vi "Configure Multi Eval Meas List Segment Bandwidth Part.vi"(0 "VISA resource name":refnum<visa-resource-name>, 1 "BWP (0)":i32, 2 "Cyclic Prefix (Normal)":i32(ring) items=["Normal", "Extended"], 3 "Start RB (0)":i32, 5 "Instance (1)":T2=1, 7 "Segment (1)":i32=1, 9 "CC (1)":T1=1, 11 "error in (no error)":errorcluster, 12 "Subcarrier Spacing (30 kHz)":i32(ring)=1 items=["15 kHz", "30 kHz", "60 kHz"], 13 "Number RB (66)":i32=66) -> (4 "VISA resource name out":refnum<visa-resource-name>, 15 "error out":errorcluster)   [LabVIEW 2020, in "Rohde&Schwarz CMWXP NR FR1 Measurement.lvlib"]
doc: "Configures basic properties of the <BWP> on carrier <cc> in segment <no>.\n\nAttribute:\nRSCMWXPNRFR1M_ATTR_MULTI_EVAL_MEAS_LIST_SEGMENT_BANDWIDTH_PART\n\nRemote-control command:\nCONFigure:NRSub:MEAS<i>:LIST:SEGMent<no>[:CC<cc>]:BWPart"
uses:
  <instrlib>/Rohde&Schwarz CMWXP NR FR1 Measurement/Rohde&Schwarz CMWXP NR FR1 Measurement.lvlib
  <instrlib>/Rohde&Schwarz CMWXP NR FR1 Measurement/Private/_Instance.ctl
  <instrlib>/Rohde&Schwarz CMWXP NR FR1 Measurement/Private/_Carrier Component.ctl
  <instrlib>/Rohde&Schwarz CMWXP NR FR1 Measurement/Private/rsidr_core.llb/rsidr_core.lvlib
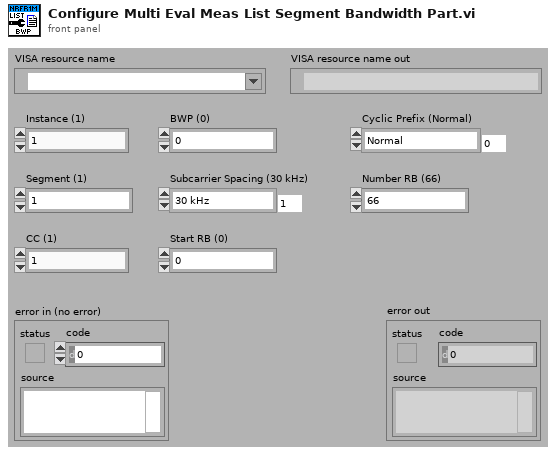
[diagram p1: front panel]
types:
  T1 = typedef "Rohde&Schwarz CMWXP NR FR1 Measurement.lvlib/_Carrier Component.ctl" = i32
  T2 = typedef "Rohde&Schwarz CMWXP NR FR1 Measurement.lvlib/_Instance.ctl" = i32
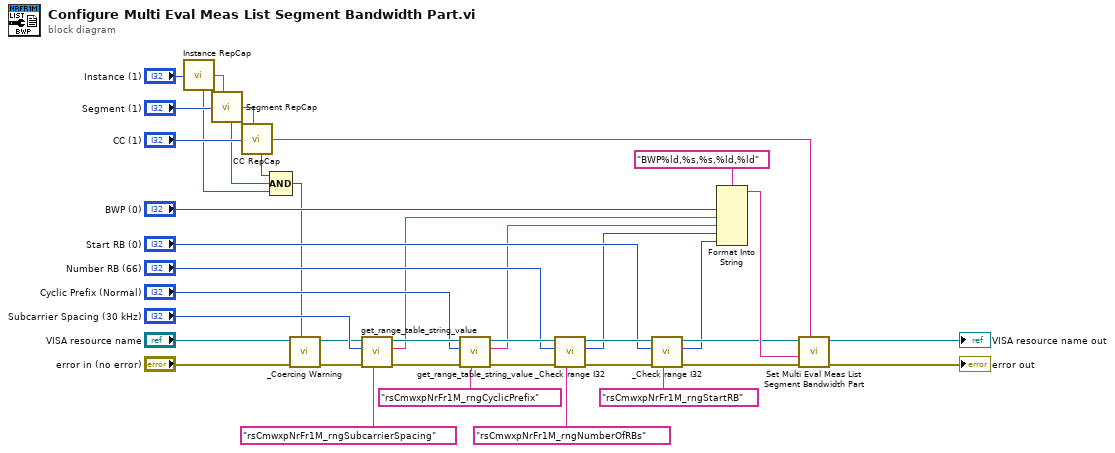
[diagram p0: block diagram]
diagram:
  n1 = call <instrlib>:"Instance RepCap.vi"("Instance In"="Instance (1)") -> ("In Range?"=w8:bool, "RepCap Identifier Out"=w33:string)  [unwired: 1 in]
  n2 = call <instrlib>:"Segment RepCap.vi"("Segment In"="Segment (1)", "RepCap String In (\"\")"=w33) -> ("In Range?"=w7:bool, "RepCap Identifier Out"=w36:string)
  n3 = call <instrlib>:"CC RepCap.vi"("CC In"="CC (1)", "RepCap String In (\"\")"=w36) -> ("In Range?"=w6:bool, "RepCap Identifier Out"=w32:string)
  n4 = Compound Arithmetic op=AND(w6, w7, w8) -> (w1:bool)
  n5 = call <instrlib>:"_Coercing Warning.vi"("In Range?"=w1, "error in (no error)"="error in (no error)", "VISA resource name"="VISA resource name") -> ("error out"=w3:errorcluster, "VISA resource name out"=w2:refnum<visa-resource-name>)  [unwired: 7 in]
  n6 = call <instrlib>:"get_range_table_string_value.vi"("Range Table ID in"="rsCmwxpNrFr1M_rngSubcarrierSpacing", "error in"=w3, "I32 input"="Subcarrier Spacing (30 kHz)", "VISA resource name"=w2) -> ("error out"=w29:errorcluster, "String Value out"=w16:string, "VISA resource name out"=w28:refnum<visa-resource-name>)  [unwired: 5 in]
  n7 = call <instrlib>:"get_range_table_string_value.vi"("Range Table ID in"="rsCmwxpNrFr1M_rngCyclicPrefix", "error in"=w29, "I32 input"="Cyclic Prefix (Normal)", "VISA resource name"=w28) -> ("error out"=w27:errorcluster, "String Value out"=w15:string, "VISA resource name out"=w26:refnum<visa-resource-name>)  [unwired: 5 in]
  n8 = call <instrlib>:"_Check range I32.vi"("Range Table Identifier"="rsCmwxpNrFr1M_rngNumberOfRBs", "error in (no error)"=w27, "I32 Value In"="Number RB (66)", "VISA resource name"=w26) -> ("error out"=w25:errorcluster, "I32 Value Out"=w14:i32, "VISA resource name out"=w24:refnum<visa-resource-name>)  [unwired: 5 in]
  n9 = call <instrlib>:"_Check range I32.vi"("Range Table Identifier"="rsCmwxpNrFr1M_rngStartRB", "error in (no error)"=w25, "I32 Value In"="Start RB (0)", "VISA resource name"=w24) -> ("error out"=w17:errorcluster, "I32 Value Out"=w13:i32, "VISA resource name out"=w18:refnum<visa-resource-name>)  [unwired: 5 in]
  n10 = Format Into String(format string="BWP%ld,%s,%s,%ld,%ld", "BWP (0)", w16, w15, w14, w13) -> (resulting string=w19:string)  [unwired: 2 in, 1 out]
  n11 = call "Set Multi Eval Meas List Segment Bandwidth Part"("Repeated Capabilities"=w32, "error in (no error)"=w17, "Multi Eval Meas List Segment Bandwidth Part ()"=w19, "instrument handle"=w18) -> ("error out"=→"error out":errorcluster, "instrument handle out"=→"VISA resource name out":refnum<visa-resource-name>)  [unwired: 6 in]
